vi "Write RT FIFO.vi"(8 "error in":errorcluster, 11 "RT Data In":refnum<class "DCM-NIVS-RT.lvclass">) -> (0 "error out":errorcluster, 3 "RT Data Out":refnum<class "DCM-NIVS-RT.lvclass">)   [LabVIEW 2016, in "DCM Engine.lvlib"]
uses:
  DCM Engine.lvlib
  Classes/DCM-NIVS-RT/DCM-NIVS-RT.lvclass
  Classes/DCM-NIVS-RT/DeviceOutFIFO Write.vi
  Classes/DCM-NIVS-RT/Device Outputs Read.vi
  Classes/DCM-NIVS-RT/DeviceOutFIFO Read.vi
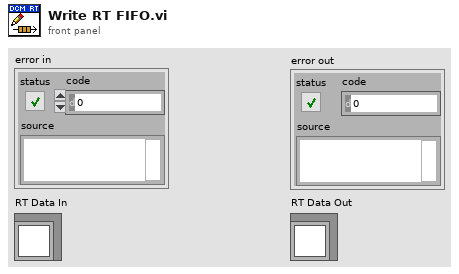
[diagram p1: front panel]
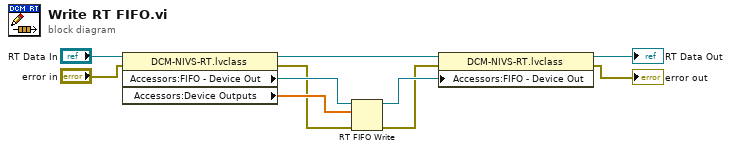
[diagram p0: block diagram]
diagram:
  n1 = property class="DCM-NIVS-RT.lvclass"(reference="RT Data In", error in="error in") -> (reference out=w5:refnum<class "DCM-NIVS-RT.lvclass">, error out=w6:errorcluster, "Accessors:FIFO - Device Out"=w7:refnum<k33>, "Accessors:Device Outputs"=w8:dbl[])
  n2 = RT FIFO Write(0:w7, 1:w8, 3:w6) -> (8:w4:refnum<k33>, 11:w3:errorcluster)  [unwired: 2 in, 2 out]
  n3 = property class="DCM-NIVS-RT.lvclass"(reference=w5, error in=w3, "Accessors:FIFO - Device Out"=w4) -> (reference out=→"RT Data Out":refnum<class "DCM-NIVS-RT.lvclass">, error out=→"error out":errorcluster)
